vi "testing.vi"() -> ()   [LabVIEW 2017]
uses:
  07d6b13e-b64f-44e3-9342-8148bbc248a8.vi
panel:
  out "send string":string
  out "send byte":u8[](array[numeric])
  out "return byte":u8[](array[numeric])
  in  "data":u8
  in  "address (first card = 1)":u8=1
  in  "command":u8
  out "error out":errorcluster
  out "read buffer":string
  in  "error in (no error)":errorcluster
  in  "VISA resource name":refnum<visa-resource-name>="COM4"
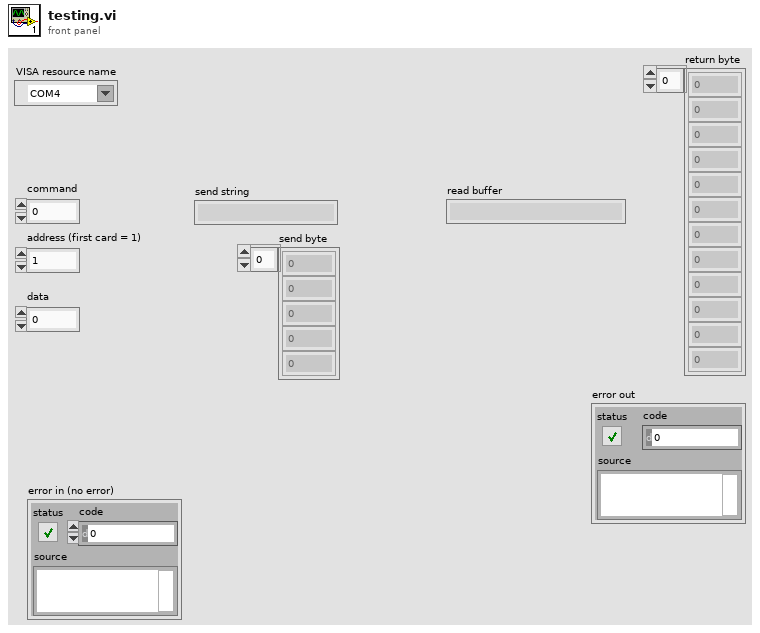
[diagram p1: front panel]
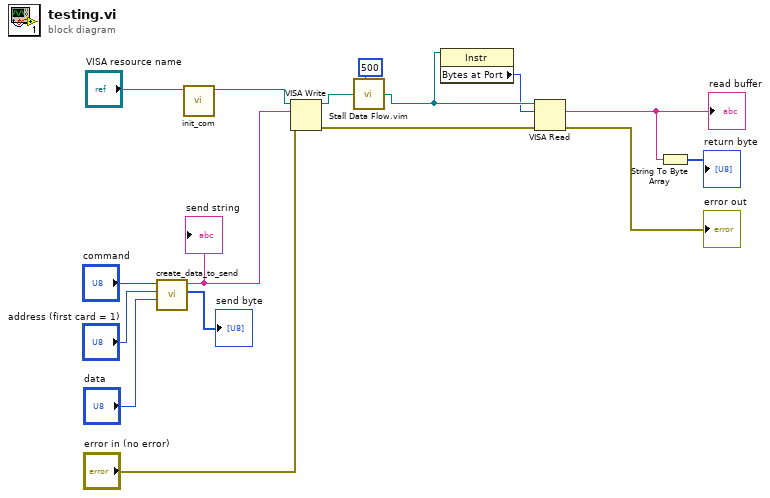
[diagram p0: block diagram]
diagram:
  n1 = call "create_data_to_send.vi"("data"="data", "address"="address (first card = 1)", "command"="command") -> ("send byte"=→"send byte":u8[], "send string"=w1:string)  [unwired: 6 in, 1 out]
  "send string" <- w1
  n2 = call "init_com.vi"("VISA Refnum in"="VISA resource name") -> ("VISA Refnum out"=w12:refnum<visa-resource-name>)  [unwired: 9 in, 1 out]
  n3 = VISA Write(VISA resource name=w12, write buffer=w1, error in (no error)="error in (no error)") -> (VISA resource name out=w11:refnum<visa-resource-name>, error out=w15:errorcluster)  [unwired: 1 out]
  n4 = call "Stall Data Flow.vim"("value in"=w11, "milliseconds to wait"=u32 500) -> ("value out"=w4:refnum<visa-resource-name>)  [unwired: 1 out]
  n5 = property class="Instr"(reference=w4) -> ("Bytes at Port"=w3:u32)  [unwired: 1 in, 2 out]
  n6 = VISA Read(VISA resource name=w4, byte count=w3, error in (no error)=w15) -> (read buffer=w5:string, error out=→"error out":errorcluster)  [unwired: 2 out]
  "read buffer" <- w5
  n7 = String To Byte Array(string=w5) -> (unsigned byte array=→"return byte":u8[])
